vi "FlexRIO7966Perf.vi"() -> ()   [LabVIEW 2013]
uses:
  Control 1.ctl
  <vilib>/Platform/TimedLoop/XDataNode/timing_clust.ctl
  <vilib>/Platform/TimedLoop/XDataNode/nitl_modes.ctl
  <vilib>/Platform/TimedLoop/XDataNode/wakeup.ctl
  Libraries/StateControl.ctl
  <vilib>/rvi/Emulation/niFpgaSctlEmulationGetInTimedLoop.vi
  <vilib>/rvi/Emulation/niFpgaEmulationReportErrorSimple.vi
  <vilib>/rvi/Emulation/niFpgaGetClockAttributes.vi
  <vilib>/rvi/Emulation/niFpgaCriticalErrorInLSC.vi
  <vilib>/rvi/FIFO/Fifo_Resource/nirvififoEmulationClearFpgaImpl.vi
  <vilib>/rvi/DataTransferAndStorage/Container/Common/niFpgaContainerGetUniqueNameForEmu.vi
  Libraries/GlobalReg.vi
  <vilib>/rvi/Emulation/niFpgaProcessEmulError.vi
  <vilib>/rvi/FIFO/Fifo_Resource/nirvififoEmulationWriteFpgaImpl.vi
  <vilib>/rvi/DataTransferAndStorage/Container/Common/niFpgaContainerExecOnDevCompGetState.vi
  <vilib>/rvi/FIFO/Fifo_Resource/nirvififoEmulationGetNumberOfElementsToReadFpgaImpl.vi
  <vilib>/rvi/interface/RandomDataEmulation/nirviRandomDataFPGAFIFO.vi
  <vilib>/rvi/interface/RandomDataEmulation/niFpgaRandomDataHandleErrors.vi
  <vilib>/rvi/eio/common/nirviEmuReportErrorAndStop.vi
  <vilib>/rvi/FIFO/Fifo_Resource/nirvififoEmulationReadFpgaImpl.vi
  <vilib>/rvi/eio/common/nirviEmuTemplateMethod_errors.vi
  <vilib>/Platform/TimedLoop/XDataNode/XDataNode.xnode
  <vilib>/rvi/DataTransferAndStorage/Container/XNode/niFpgaContainer.xnode
  <vilib>/rvi/FIFO/Fifo_Resource/nirvififoEmulationClear.vi
  <vilib>/rvi/FIFO/Fifo_Resource/nirvififoEmulationWrite.vi
  <vilib>/rvi/FIFO/Fifo_Resource/niFpgaFifoEmulationRefIn.vi
  <vilib>/rvi/interface/RandomDataEmulation/nirviRandomDataFpgaReadWriteTemplate.vi
  <vilib>/eio/EIONode/EIONode.xnode
  <vilib>/Platform/TimedLoop/XDataNode/XDNodeRunTimeDep.lvlib
panel:
  in  "Tab Control":T1(tab)=enum."Data Acquisition"
  out "Platform":enum8{"FlexRIO", "cRIO", "RSeries"}(ring)
  out "FPGAVIversion":u8[](array[numeric])=[1, 1]
  out "InitDone":bool
  out "RIOAdapterCorrect":bool
  out "Fref":u32=125000000
  out "DevQualityStatus":u8
  out "DevTemp":i16=-10244
  out "DevProfile":u8 format="%x"
  in  "DAQStartStop":bool
  in  "DebugMode":bool
  out "Expected IO Module ID":u32 format="%x"
  out "InsertedIOModule ID":u32
  out "DMATtoHOSTNCh":T2[](array[typedef])=[4]
  out "DMATtoHOSTFrameType":u8[](array[numeric])
  out "DMATtoHOSTSampleSize":u8[](array[numeric])=[2]
  out "DMATtoHOSTBlockNWords":u16[](array[numeric])=[4096]
  in  "DMATtoHOSTSamplingRate0":u16=10000
  in  "DMATtoHOSTEnable0":bool
  out "DMATtoHOSTOverflows":u16
  out "auxAI5":i32
  out "auxAI4":i32
  out "auxAI3":i32
  out "auxAI2":i32
  out "auxAI1":i32
  out "auxAI0":i32
  in  "auxAO5":i32
  in  "auxAO4":i32
  in  "auxAO3":i32
  in  "auxAO2":i32
  in  "auxAO1":i32
  in  "auxAO0":i32
  out "auxDI5":bool
  out "auxDI4":bool
  out "auxDI3":bool
  out "auxDI2":bool
  out "auxDI1":bool
  out "auxDI0":bool
  in  "auxDO3":bool
  in  "auxDO4":bool
  in  "auxDO5":bool
  in  "auxDO2":bool
  in  "auxDO1":bool
  in  "auxDO0":bool
  in  "SGUpdateRate0":u32=40
  in  "SGPhase0":u32
  in  "SGFreq0":u32=100000
  in  "SGAmp0":u16
  in  "AO0":i32
  out "auxAI9":i32
  out "SGNo":u8=2 format="%x"
  out "auxAI10":i32
  in  "SGSignalType1":u8
  in  "SGAmp1":u16
  in  "SGPhase1":u32
  in  "SGFreq1":u32=100000
  in  "SGUpdateRate1":u32=40
  in  "AO1":i32
  in  "AOEnable1":bool
  out "SGFref0":u32=100000000
  out "SGFref1":u32=100000000
  in  "AOEnable0":bool
  in  "SGSignalType0":u8
  out "auxDI6":bool
  # "Inputs"
  # "Aux \nDigital Inputs"
  # "Aux \nAnalog Inputs"
  # "Digital Inputs"
  # "Outputs"
  # "Number of WF gen"
  # "Analog Outputs"
  # "Aux Digital \nOutput"
  # "Digital\nOutputs"
  # "Aux Analog \nOutput"
  # "Signal Generator 1"
  # "Signal Generator 0"
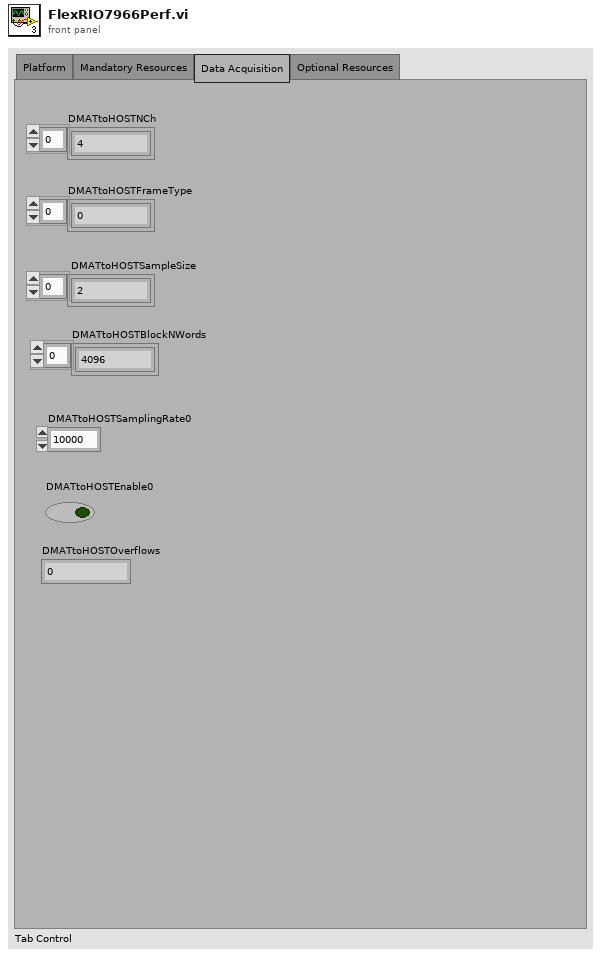
[diagram p1: front panel]
types:
  T1 = enum32{"Platform", "Mandatory Resources", "Data Acquisition", "Optional Resources"}
  T2 = typedef "Control 1.ctl" = u16
  T3 = typedef "XDNodeRunTimeDep.lvlib/timing_clust.ctl" = cluster{"Expected End [f-1]":u64, "Actual End [f-1]":u64, "Finished Late? [f-1]":bool, "Expected End [i-1]":u64, "Actual End [i-1]":u64, "Finished Late? [i-1]":bool, "Expected Start [i]":u64, "Actual Start [i]":u64, "Expected Start [f]":u64, "Actual Start [f]":u64, "Source Name":string, "Structure Name":string, "Period":i64, "Deadline":i64, "Offset":i64, "Start":i64, "Priority":i32, "Timeout":i32, "Mode":T4, "Wakeup Reason":T5, "Error":errorcluster, "Source Type":string, "Secondary Source Type":string, "Global End Time":u64, "Global Start Time":u64, "Frame Duration":u64, "Iteration Duration":u64, "Assigned CPU":i32, "I/O Scan Engine Mode":u32}
  T4 = typedef "XDNodeRunTimeDep.lvlib/nitl_modes.ctl" = enum32{"No Change", "Process missed periods, maintain original phase", "Discard missed periods, maintain original phase", "Process missed periods, ignore original phase", "Discard missed periods, ignore original phase"}
  T5 = typedef "XDNodeRunTimeDep.lvlib/wakeup.ctl" = enum32{"Normal", "Aborted", "Asynchronous wakeup", "Timing source error", "Timed loop error", "Timeout"}
  T6 = typedef "StateControl.ctl" = enum16{"Idle", "Acq"}
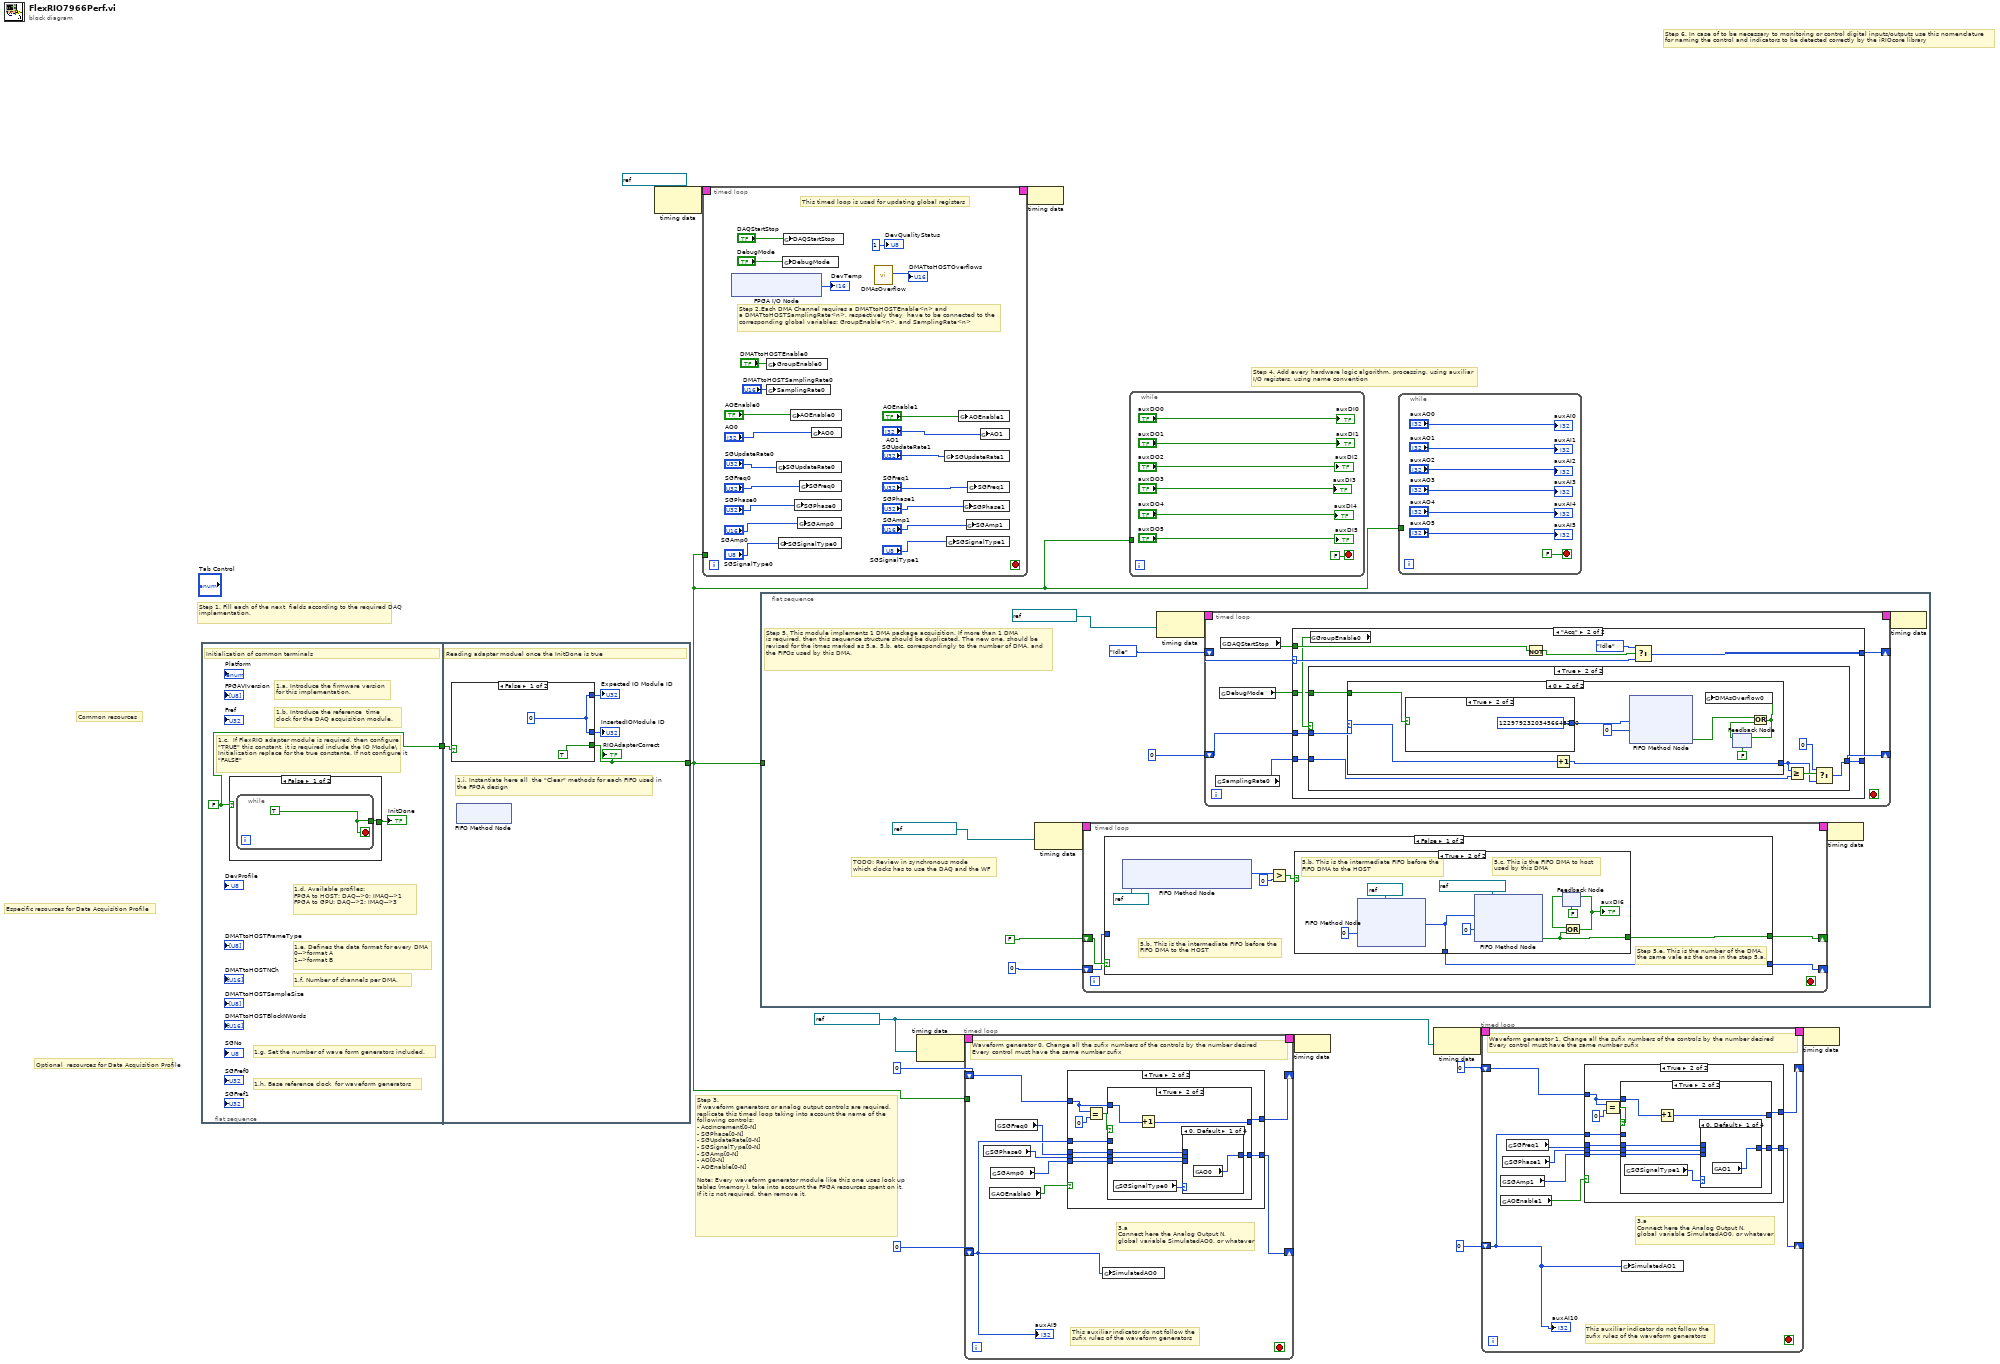
[diagram p0: block diagram]
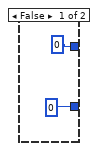
[diagram p2: hidden frame]
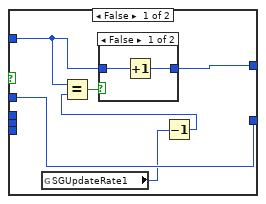
[diagram p3: hidden frame]
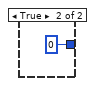
[diagram p4: hidden frame]
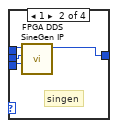
[diagram p5: hidden frame]
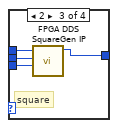
[diagram p6: hidden frame]
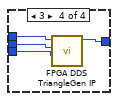
[diagram p7: hidden frame]
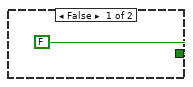
[diagram p8: hidden frame]
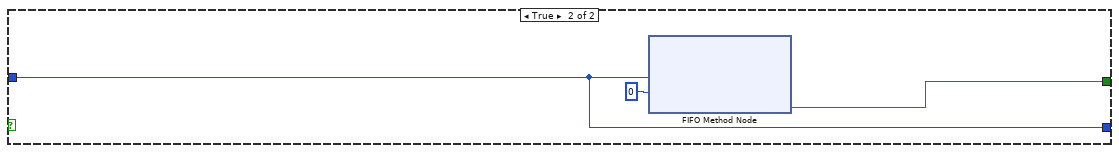
[diagram p9: hidden frame]
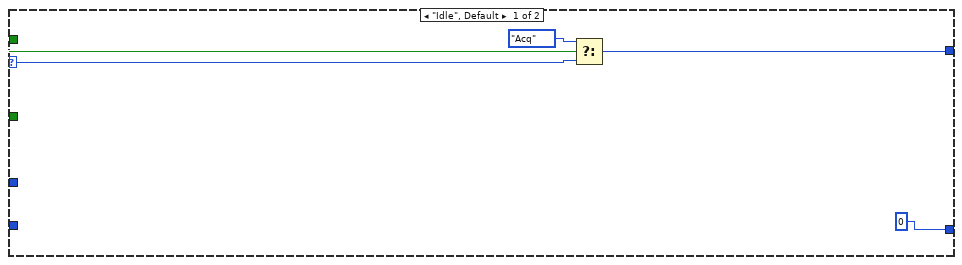
[diagram p10: hidden frame]
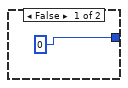
[diagram p11: hidden frame]
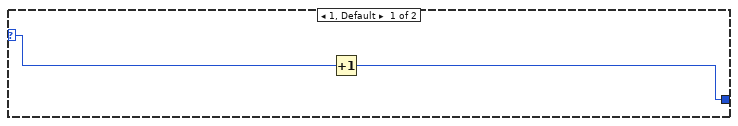
[diagram p12: hidden frame]
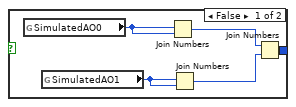
[diagram p13: hidden frame]
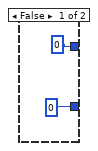
[diagram p14: hidden frame]
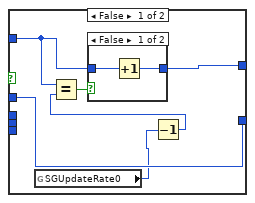
[diagram p15: hidden frame]
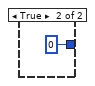
[diagram p16: hidden frame]
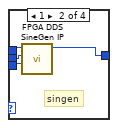
[diagram p17: hidden frame]
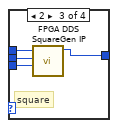
[diagram p18: hidden frame]
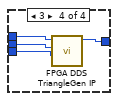
[diagram p19: hidden frame]
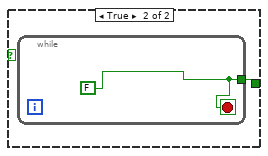
[diagram p20: hidden frame]
diagram:
  w1 = refnum<k21> "100 MHz Clock" ("Source Name")
  # "Step 6. In case of to be necessary to monitoring or control digital inputs/outputs use this nomenclature\nfor naming the control and indicators to be detected correctly by the iRIOcore library"
  # "Optional  resources for Data Acquisition Profile"
  # "Especific resources for Data Acquisition Profile"
  # "Common resources"
  # "Step 4. Add every hardware logic algorithm, processing, using auxiliar \nI/O registers, using name convention"
  # "Step 3.\nIf waveform generators or analog output controls are required,\nreplicate this timed loop taking into account the name of the \nfollowing controls:\n- AccIncrement[0-N]\n- SGPhase[0-N]\n- SGUpdateRate[0-N]\n- SGSignalType[0-N]\n- SGAmp[0-N]\n- AO[0-N]\n- AOEnable[0-N]\n\nNote: Every waveform generator module like this one uses look up tables (memory), take into account the FPGA resources spent on it.  If it is not required, then remove it."
  # "Step 1. Fill each of the next  fields according to the required DAQ implementation."
  n1 = flat-sequence {
    tunnel: [w15] -> w14
    tunnel: [w22] -> w6
    tunnel: w14 -> [w21]
    frame #0 {
      w15 = FALSE
      # "1.h. Base reference clock  for waveform generators"
      # "1.e. Defines the data format for every DMA\n0-->format A\n1-->format B"
      # "1.c.  If FlexRIO adapter module is required, then configure \"TRUE\" this constant, it is required include the IO Module\\Initialization replace for the true constante. If not configure it \"FALSE\""
      # "1.a. Introduce the firmware version \nfor this implementation."
      # "1.b. Introduce the reference  time \nclock for the DAQ acquisition module."
      # "1.g. Set the number of wave form generators included."
      # "1.f. Number of channels per DMA."
      # "1.d. Available profiles: \nFPGA to HOST: DAQ-->0; IMAQ-->1\nFPGA to GPU: DAQ-->2; IMAQ-->3"
      # "Initialization of common terminals"
      n2 = case shown="False" w15 {
        tunnel: [w17 w19] -> w16
        frame False {
          n3 = while {
            tunnel: [w18] -> w17
            stop <- w18 stop-if-true
            w18 = TRUE
          }
        }
        frame True {
          n4 = while {
            tunnel: [w20] -> w19
            stop <- w20 stop-if-true
            w20 = FALSE
          }
        }
      }
      "InitDone" <- w16
    }
    frame #1 {
      # "1.i. Instantiate here all  the \"Clear\" methods for each FIFO used in the FPGA design"
      # "Reading adapter moduel once the InitDone is true"
      n5 = case shown="False" w21 {
        tunnel: [TRUE w29] -> w22
        tunnel: [w26 w28] -> w24
        tunnel: [w26 w27] -> w23
        frame False {
          w26 = u32 0
        }
        frame True {
          n6 = xnode "FPGA I/O Node"() -> ("Expected IO Module ID"=w28:u32)  [unwired: 1 in, 1 out]
          n7 = xnode "FPGA I/O Node"() -> ("Inserted IO Module ID"=w27:u32)  [unwired: 1 in, 1 out]
          n8 = Equal?(x=w28, y=w27) -> (x = y?=w29:bool)
        }
      }
      "Expected IO Module ID" <- w24
      "InsertedIOModule ID" <- w23
      "RIOAdapterCorrect" <- w22
      n9 = xnode ("FIFO Method Node")() -> ()  [unwired: 1 in, 1 out]
    }
  }
  n10 = node-c288(refnum<k21> "100 MHz Clock" ("Source Name")) -> (w9:T3)
  n11 = timed-loop {
    timing: w9 -> [_]
    timing-out: [_] -> w8
    tunnel: w6 -> [_]
    stop <- _ stop-if-true
    # "This timed loop is used for updating global registers"
    # "Step 2.Each DMA Channel requires a DMATtoHOSTEnable<n> and\na DMATtoHOSTSamplingRate<n>, respectively they  have to be connected to the\ncorresponding global variables: GroupEnable<n>, and SamplingRate<n>"
    n12 = xnode "FPGA I/O Node"() -> ("Device Temperature"=→"DevTemp":i16)  [unwired: 1 in, 1 out]
    n13 = global write "GlobalReg.vi" "GroupEnable0"("DMATtoHOSTEnable0") -> ()
    n14 = global write "GlobalReg.vi" "SamplingRate0"("DMATtoHOSTSamplingRate0") -> ()
    n15 = global write "GlobalReg.vi" "SGUpdateRate0"("SGUpdateRate0") -> ()
    n16 = global write "GlobalReg.vi" "SGSignalType0"("SGSignalType0") -> ()
    n17 = global write "GlobalReg.vi" "DebugMode"("DebugMode") -> ()
    n18 = global write "GlobalReg.vi" "DAQStartStop"("DAQStartStop") -> ()
    n19 = global write "GlobalReg.vi" "AOEnable0"("AOEnable0") -> ()
    n20 = global write "GlobalReg.vi" "SGPhase0"("SGPhase0") -> ()
    n21 = global write "GlobalReg.vi" "SGAmp0"("SGAmp0") -> ()
    n22 = global write "GlobalReg.vi" "SGFreq0"("SGFreq0") -> ()
    n23 = global write "GlobalReg.vi" "AO0"("AO0") -> ()
    n24 = call "DMAsOverflow.vi"() -> ("DMAsOverFlow"=→"DMATtoHOSTOverflows":u16)  [unwired: 11 in]
    n25 = global write "GlobalReg.vi" "SGUpdateRate1"("SGUpdateRate1") -> ()
    n26 = global write "GlobalReg.vi" "SGSignalType1"("SGSignalType1") -> ()
    n27 = global write "GlobalReg.vi" "AOEnable1"("AOEnable1") -> ()
    n28 = global write "GlobalReg.vi" "SGPhase1"("SGPhase1") -> ()
    n29 = global write "GlobalReg.vi" "SGAmp1"("SGAmp1") -> ()
    n30 = global write "GlobalReg.vi" "SGFreq1"("SGFreq1") -> ()
    n31 = global write "GlobalReg.vi" "AO1"("AO1") -> ()
    "DevQualityStatus" <- u8 1 ("DevQualityStatus")
  }
  n32 = flat-sequence {
    tunnel: w6 -> [_]
    frame #0 {
      # "TODO: Review in synchronous mode \nwhich clocks has to use the DAQ and the WF"
      # "Step 5. This module implements 1 DMA package acquisition. If more than 1 DMA \nis required, then this sequence structure should be duplicated. The new one, should be \nrevised for the itmes marked as 5.a, 5.b, etc. correspondingly to the number of DMA, and \nthe FIFOs used by this DMA."
      n33 = node-c288(refnum<k21> "100 MHz Clock" ("Source Name")) -> (w60:T3)
      n34 = timed-loop {
        timing: w60 -> [_]
        timing-out: [_] -> w59
        shift-right: [w66] -> _
        shift-left: FALSE ("Timed Out?") -> [w65]
        shift-right: [w64] -> _
        shift-left: u64 0 -> [w63]
        stop <- _ stop-if-true
        n35 = case shown="False" w65 {
          tunnel: [w69 w84] -> w66
          tunnel: [w67 w83] -> w64
          tunnel: w63 -> [_ w83]
          frame False {
            # "Step 5.e. This is the number of the DMA,\nthe same vale as the one in the step 5.a."
            # "5.b. This is the intermediate FIFO before the \nFIFO DMA to the HOST"
            n36 = xnode ("FIFO Method Node")("FIFO In"=refnum<k21> "FIFO0" ("IntermediateFIFO")) -> ("Number of Elements to Read"=w72:u32)  [unwired: 1 out]
            n37 = Greater?(x=w72, y=u32 0) -> (0:w70:bool)
            n38 = case shown="True" w70 {
              tunnel: [FALSE ("Timed Out?") w77] -> w69
              tunnel: [_ w78] -> w67
              frame False {
              }
              frame True {
                # "5.c. This is the FIFO DMA to host \nused by this DMA"
                # "5.b. This is the intermediate FIFO before the \nFIFO DMA to the HOST"
                n39 = xnode ("FIFO Method Node")("Timeout"=0, "FIFO In"=refnum<k21> "FIFO0" ("IntermediateFIFO")) -> ("Element"=w78:u64)  [unwired: 2 out]
                n40 = xnode ("FIFO Method Node")("Element"=w78, "Timeout"=0, "FIFO In"=refnum<k21> "DMATtoHOST0") -> ("Timed Out?"=w77:bool)  [unwired: 1 out]
                n41 = feedback #1(FALSE) -> (w76:bool)
                n42 = Or(x=w76, y=w77) -> (x .or. y?=w75:bool)
                "auxDI6" <- w75
                n43 = feedback-in #1(w75) -> ()
              }
            }
          }
          frame True {
            n44 = xnode ("FIFO Method Node")("Element"=w83, "Timeout"=0) -> ("Timed Out?"=w84:bool)  [unwired: 1 in, 1 out]
          }
        }
      }
      n45 = node-c288(refnum<k21> "100 MHz Clock" ("Source Name")) -> (w62:T3)
      n46 = timed-loop {
        timing: w62 -> [_]
        timing-out: [_] -> w61
        shift-right: [w97] -> _
        shift-left: StateControl."Idle" ("Enum") -> [w98]
        shift-right: [w93] -> _
        shift-left: i16 0 -> [w94]
        stop <- _ stop-if-true
        n47 = global read "GlobalReg.vi" "SamplingRate0"() -> (w95:u16)
        n48 = global read "GlobalReg.vi" "DebugMode"() -> (w92:bool)
        n49 = global read "GlobalReg.vi" "DAQStartStop"() -> (w96:bool)
        n50 = case shown="\"Acq\"" w98 {
          selector: w98 -> [w101 w112]
          tunnel: w96 -> [w103 w109]
          tunnel: [w100 w111] -> w97
          tunnel: w95 -> [_ w107]
          tunnel: w94 -> [_ w106]
          tunnel: [i16 0 w105] -> w93
          tunnel: w92 -> [_ w104]
          frame "Idle", Default {
            n51 = Select(t=StateControl."Acq" ("Enum"), s=w103, f=w101) -> (s? t:f=w100:T6)
          }
          frame "Acq" {
            n52 = global read "GlobalReg.vi" "GroupEnable0"() -> (w108:bool)
            n53 = case shown="True" w108 {
              tunnel: w107 -> [_ w120]
              tunnel: w106 -> [_ w121]
              tunnel: [i16 0 w117] -> w105
              tunnel: w104 -> [_ w115]
              frame False {
              }
              frame True {
                n54 = case shown="0" w121 {
                  selector: w121 -> [w123 w126]
                  tunnel: [w122 w125] -> w116
                  tunnel: w115 -> [_ w124]
                  frame 1, Default {
                    n55 = Increment(x=w123) -> (x+1=w122:u16)
                  }
                  frame 0 {
                    n56 = case shown="True" w124 {
                      tunnel: [w133 u64 12297923203456648260] -> w132
                      frame False {
                        n57 = global read "GlobalReg.vi" "SimulatedAO0"() -> (w137:i16)
                        n58 = global read "GlobalReg.vi" "SimulatedAO1"() -> (w136:i16)
                        n59 = Join Numbers(hi=w137, lo=w137) -> ((hi.lo)=w135:u32)
                        n60 = Join Numbers(hi=w136, lo=w136) -> ((hi.lo)=w134:u32)
                        n61 = Join Numbers(hi=w135, lo=w134) -> ((hi.lo)=w133:u64)
                      }
                      frame True {
                      }
                    }
                    n62 = Increment(x=w126) -> (x+1=w125:u16)
                    n63 = xnode ("FIFO Method Node")("Element"=w132, "Timeout"=0) -> ("Timed Out?"=w130:bool)  [unwired: 1 in, 1 out]
                    n64 = feedback #2(FALSE) -> (w128:bool)
                    n65 = Or(x=w130, y=w128) -> (x .or. y?=w129:bool)
                    n66 = global write "GlobalReg.vi" "DMAsOverflow0"(w129) -> ()
                    n67 = feedback-in #2(w129) -> ()
                  }
                }
                n68 = Greater Or Equal?(x=w116, y=w120) -> (x >= y?=w119:bool)
                n69 = Select(t=u16 0, s=w119, f=w116) -> (s? t:f=w117:u16)
              }
            }
            n70 = Not(x=w109) -> (.not. x?=w110:bool)
            n71 = Select(t=StateControl."Idle" ("Enum"), s=w110, f=w112) -> (s? t:f=w111:T6)
          }
        }
      }
      n72 = node-c288(w59) -> ()
      n73 = node-c288(w61) -> ()
    }
  }
  n74 = node-c288(w1) -> (w13:T3)
  n75 = timed-loop {
    shift-right: [w152] -> _
    shift-left: i16 0 ("Signal Value") -> [w149]
    timing: w13 -> [_]
    timing-out: [_] -> w12
    shift-right: [w150] -> _
    shift-left: u32 0 -> [w151]
    tunnel: w6 -> [_]
    stop <- _ stop-if-true
    # "This auxiliar indicator do not follow the \nsufix rules of the waveform generators"
    # "3.a\nConnect here the Analog Output N,\nglobal variable SimulatedAO0, or whatever"
    # "Waveform generator 0. Change all the sufix numbers of the controls by the number desired\nEvery control must have the same number sufix"
    n76 = global read "GlobalReg.vi" "SGPhase0"() -> (w147:u32)
    n77 = global read "GlobalReg.vi" "AOEnable0"() -> (w145:bool)
    n78 = global read "GlobalReg.vi" "SGAmp0"() -> (w146:u16)
    n79 = global read "GlobalReg.vi" "SGFreq0"() -> (w148:u32)
    n80 = case shown="True" w145 {
      tunnel: w148 -> [_ w163]
      tunnel: w147 -> [_ w162]
      tunnel: w146 -> [_ w161]
      tunnel: [i16 0 w160] -> w152
      tunnel: w151 -> [_ w157]
      tunnel: [u32 0 w156] -> w150
      tunnel: w149 -> [_ w155]
      frame False {
      }
      frame True {
        n81 = Equal?(x=w157, y=u32 0) -> (x = y?=w159:bool)
        n82 = case shown="True" w159 {
          tunnel: w163 -> [_ w179]
          tunnel: w162 -> [_ w178]
          tunnel: w161 -> [_ w177]
          tunnel: [w168 w176] -> w160
          tunnel: w157 -> [w167 w175]
          tunnel: [w169 w174] -> w156
          tunnel: w155 -> [w168 _]
          frame False {
            n83 = global read "GlobalReg.vi" "SGUpdateRate0"() -> (w164:u32)
            n84 = Decrement(x=w164) -> (x-1=w165:u32)
            n85 = Equal?(x=w167, y=w165) -> (x = y?=w166:bool)
            n86 = case shown="False" w166 {
              tunnel: w167 -> [w171 _]
              tunnel: [w170 u32 0] -> w169
              frame False {
                n87 = Increment(x=w171) -> (x+1=w170:u32)
              }
              frame True {
              }
            }
          }
          frame True {
            n88 = global read "GlobalReg.vi" "SGSignalType0"() -> (w173:u8)
            n89 = Increment(x=w175) -> (x+1=w174:u32)
            n90 = case shown="0, Default" w173 {
              tunnel: w179 -> [_ w184 w188 w192]
              tunnel: w178 -> [_ w183 w187 w191]
              tunnel: w177 -> [_ w182 w186 w190]
              tunnel: [w180 w181 w185 w189] -> w176
              frame 0, Default {
                n91 = global read "GlobalReg.vi" "AO0"() -> (w180:i32)
              }
              frame 1 {
                # "singen"
                n92 = call "FPGA DDS SineGen IP.vi"("Signal Amplitude (x 2^15)"=w182, "Phase Shift"=w183, "Accumulator Increment"=w184) -> ("Signal Value"=w181:i16)  [unwired: 7 in, 1 out]
              }
              frame 2 {
                # "square"
                n93 = call "FPGA DDS SquareGen IP.vi"("Signal Amplitude (x 2^15)"=w186, "Phase Shift"=w187, "Accumulator Increment"=w188) -> ("Signal Value"=w185:i16)  [unwired: 7 in, 1 out]
              }
              frame 3 {
                n94 = call "FPGA DDS TriangleGen IP.vi"("Signal Amplitude (x 2^15)"=w190, "Phase Shift"=w191, "Accumulator Increment"=w192) -> ("Signal Value"=w189:i16)  [unwired: 7 in, 1 out]
              }
            }
          }
        }
      }
    }
    n95 = global write "GlobalReg.vi" "SimulatedAO0"(w149) -> ()
    "auxAI9" <- w149
  }
  n96 = node-c288(w8) -> ()
  n97 = while {
    tunnel: w6 -> [_]
    stop <- FALSE stop-if-true
    "auxDI0" <- "auxDO0"
    "auxDI1" <- "auxDO1"
    "auxDI2" <- "auxDO2"
    "auxDI3" <- "auxDO3"
    "auxDI4" <- "auxDO4"
    "auxDI5" <- "auxDO5"
  }
  n98 = node-c288(w12) -> ()
  n99 = while {
    tunnel: w6 -> [_]
    stop <- FALSE stop-if-true
    "auxAI0" <- "auxAO0"
    "auxAI1" <- "auxAO1"
    "auxAI2" <- "auxAO2"
    "auxAI3" <- "auxAO3"
    "auxAI4" <- "auxAO4"
    "auxAI5" <- "auxAO5"
  }
  n100 = node-c288(w1) -> (w5:T3)
  n101 = timed-loop {
    shift-right: [w216] -> _
    shift-left: i16 0 ("Signal Value") -> [w209]
    timing: w5 -> [_]
    timing-out: [_] -> w4
    shift-right: [w214] -> _
    shift-left: u32 0 -> [w215]
    stop <- _ stop-if-true
    # "This auxiliar indicator do not follow the \nsufix rules of the waveform generators"
    # "3.a\nConnect here the Analog Output N,\nglobal variable SimulatedAO0, or whatever"
    # "Waveform generator 1. Change all the sufix numbers of the controls by the number desired\nEvery control must have the same number sufix"
    n102 = global read "GlobalReg.vi" "SGAmp1"() -> (w211:u16)
    n103 = global read "GlobalReg.vi" "AOEnable1"() -> (w210:bool)
    n104 = global read "GlobalReg.vi" "SGPhase1"() -> (w212:u32)
    n105 = global read "GlobalReg.vi" "SGFreq1"() -> (w213:u32)
    n106 = case shown="True" w210 {
      tunnel: w213 -> [_ w227]
      tunnel: w212 -> [_ w226]
      tunnel: w211 -> [_ w225]
      tunnel: [i16 0 w224] -> w216
      tunnel: w215 -> [_ w221]
      tunnel: [u32 0 w220] -> w214
      tunnel: w209 -> [_ w219]
      frame False {
      }
      frame True {
        n107 = Equal?(x=w221, y=u32 0) -> (x = y?=w223:bool)
        n108 = case shown="True" w223 {
          tunnel: w227 -> [_ w243]
          tunnel: w226 -> [_ w242]
          tunnel: w225 -> [_ w241]
          tunnel: [w232 w240] -> w224
          tunnel: w221 -> [w231 w239]
          tunnel: [w233 w238] -> w220
          tunnel: w219 -> [w232 _]
          frame False {
            n109 = global read "GlobalReg.vi" "SGUpdateRate1"() -> (w228:u32)
            n110 = Decrement(x=w228) -> (x-1=w229:u32)
            n111 = Equal?(x=w231, y=w229) -> (x = y?=w230:bool)
            n112 = case shown="False" w230 {
              tunnel: w231 -> [w235 _]
              tunnel: [w234 u32 0] -> w233
              frame False {
                n113 = Increment(x=w235) -> (x+1=w234:u32)
              }
              frame True {
              }
            }
          }
          frame True {
            n114 = global read "GlobalReg.vi" "SGSignalType1"() -> (w237:u8)
            n115 = Increment(x=w239) -> (x+1=w238:u32)
            n116 = case shown="0, Default" w237 {
              tunnel: w243 -> [_ w248 w252 w256]
              tunnel: w242 -> [_ w247 w251 w255]
              tunnel: w241 -> [_ w246 w250 w254]
              tunnel: [w244 w245 w249 w253] -> w240
              frame 0, Default {
                n117 = global read "GlobalReg.vi" "AO1"() -> (w244:i32)
              }
              frame 1 {
                # "singen"
                n118 = call "FPGA DDS SineGen IP.vi"("Signal Amplitude (x 2^15)"=w246, "Phase Shift"=w247, "Accumulator Increment"=w248) -> ("Signal Value"=w245:i16)  [unwired: 7 in, 1 out]
              }
              frame 2 {
                # "square"
                n119 = call "FPGA DDS SquareGen IP.vi"("Signal Amplitude (x 2^15)"=w250, "Phase Shift"=w251, "Accumulator Increment"=w252) -> ("Signal Value"=w249:i16)  [unwired: 7 in, 1 out]
              }
              frame 3 {
                n120 = call "FPGA DDS TriangleGen IP.vi"("Signal Amplitude (x 2^15)"=w254, "Phase Shift"=w255, "Accumulator Increment"=w256) -> ("Signal Value"=w253:i16)  [unwired: 7 in, 1 out]
              }
            }
          }
        }
      }
    }
    n121 = global write "GlobalReg.vi" "SimulatedAO1"(w209) -> ()
    "auxAI10" <- w209
  }
  n122 = node-c288(w4) -> ()
